vi "SLSC Convert ENUM Value to ENUM String.vi"(11 "Enums":T2[](array[typedef])) -> (2 "Cluster Enums":T1(array[cluster]), 3 "String Enums":cluster{"name":string, "string enums":string}[](array[cluster]))   [LabVIEW 2017, in "SLSC Tree Control.lvlib"]
doc: "Converts the ENUM datatype into ENUM strings used in the SLSC Output Tree control."
uses:
  SLSC Tree Control.lvlib
  SLSC EDS API/JSON parsing/enum.ctl
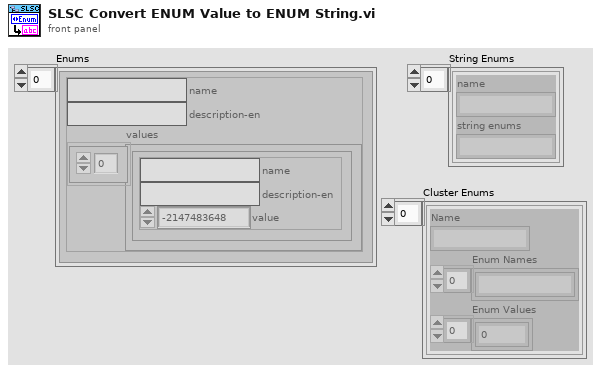
[diagram p1: front panel]
types:
  T1 = cluster{"Name":string, "Enum Names":string[], "Enum Values":i32[]}[]
  T2 = typedef "enum.ctl" = cluster{"name":string, "description-en":string, "values":cluster{"name":string, "description-en":string, "value":i32}[]}
  T3 = cluster{"name":string, "description-en":string, "value":i32}[]
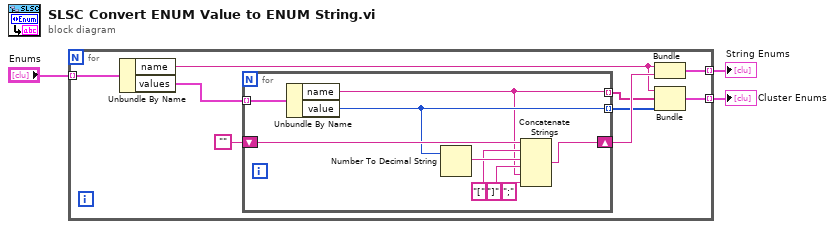
[diagram p0: block diagram]
diagram:
  n1 = for {
    tunnel: "Enums" -> [w12] mode=indexing
    tunnel: [w8] -> w3 mode=indexing
    tunnel: [w5] -> w1 mode=indexing
    n2 = Unbundle By Name(w12) -> ("name"=w4:string, "values"=w11:T3)
    n3 = for {
      tunnel: w11 -> [w15] mode=indexing
      shift-right: [w21] -> w9
      shift-left: "" -> [w20]
      tunnel: [w14] -> w6 mode=indexing
      tunnel: [w13] -> w7 mode=indexing
      n4 = Unbundle By Name(w15) -> ("name"=w13:string, "value"=w14:i32)
      n5 = Number To Decimal String(number=w14) -> (decimal integer string=w19:string)  [unwired: 1 in]
      n6 = Concatenate Strings(w20, "[" ("string"), w19, "]" ("string"), w13, ";" ("string")) -> (w21:string)
    }
    n7 = Bundle("name"=w4, w9) -> (w8:cluster{"name":string, string})  [unwired: 1 in]
    n8 = Bundle("name"=w4, w7, w6) -> (w5:cluster{"name":string, string[], i32[]})  [unwired: 1 in]
  }
  "String Enums" <- w3
  "Cluster Enums" <- w1
